vi "Generate Data.vi"(8 "error in":errorcluster, 11 "Number of Channels":i32) -> (0 "error out":errorcluster, 2 "Power Spectrum Data":waveform(dbl)[](graph) caption="Power Spectrum", 3 "Waveform Chart":waveform(dbl)[](graph))   [LabVIEW 2010]
uses:
  <vilib>/express/express analysis/Spectral/XNode/ExpressSpectralMeasurementsBlockNode.xnode
  Instance           3 21Saved   Generate Data .vi
  Instance           4 21Saved   Generate Data .vi
  Instance           1 21Saved   Generate Data .vi
  <vilib>/express/express analysis/Spectral/Block/exnSpectralBlock spectral measurements power poly.vi
  <vilib>/express/express analysis/Spectral/Block/exnSpectralBlock spectral measurements power DDT.vi
panel:
  in  "Empty":dynamicdata(waveform)
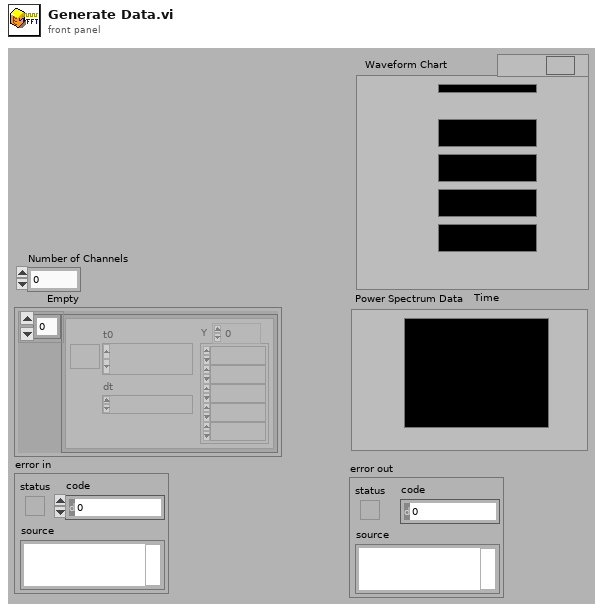
[diagram p1: front panel]
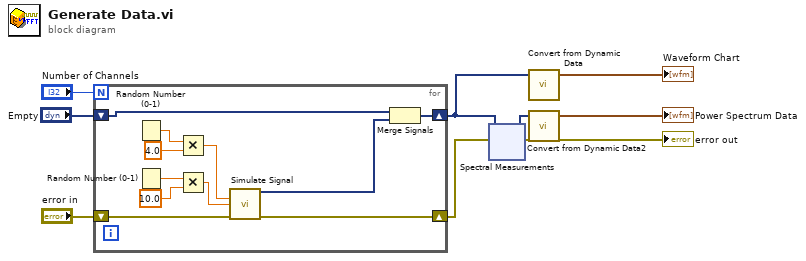
[diagram p0: block diagram]
diagram:
  n1 = for {
    N: "Number of Channels" -> [_]
    shift-right: [w13] -> w7
    shift-left: "error in" -> [w17]
    shift-right: [w16] -> w4
    shift-left: "Empty" -> [w14]
    n2 = Random Number (0-1)() -> (number: 0 to 1=w11:dbl)
    n3 = Random Number (0-1)() -> (number: 0 to 1=w20:dbl)
    n4 = Multiply(x=w11, y=4.0) -> (x*y=w10:dbl)
    n5 = Multiply(x=w20, y=10.0) -> (x*y=w18:dbl)
    n6 = call "Simulate Signal"("Frequency"=w10, "Amplitude"=w18, "error in (no error)"=w17) -> ("Sine"=w15:dynamicdata, "error out"=w13:errorcluster)  [unwired: 11 in]
    n7 = Merge Signals(w14, w15) -> (w16:dynamicdata)
  }
  n8 = xnode "Spectral Measurements"("Signals"=w4, "error in (no error)"=w7) -> ("Power Spectrum"=w2:dynamicdata, "error out"=→"error out":errorcluster)
  n9 = call "Convert from Dynamic Data"("Dynamic Data Type"=w4) -> ("Array of Waveform"=→"Waveform Chart":waveform(dbl)[])  [unwired: 3 in]
  n10 = call "Convert from Dynamic Data2"("Dynamic Data Type"=w2) -> ("Array of Waveform"=→"Power Spectrum Data":waveform(dbl)[])  [unwired: 3 in]
